vi "Write Reader.vi"(8 "error in (no error)":errorcluster, 10 "BaseReader.lvclass":refnum<class "BaseReader.lvclass">, 11 "BaseDriver in":refnum<class "BaseDriver.lvclass">) -> (0 "error out":errorcluster, 3 "BaseDriver out":refnum<class "BaseDriver.lvclass">)   [LabVIEW 2013, in "BaseDriver.lvclass"]
doc: "The Reader is the object that will perform the actual writing and reading from the remote destination. It should be a child of the BaseReader class and contains overloadded methods for writing to whatever destination it communicates with, such as a serial line or a TCP/IP connection"
uses:
  BaseDriver.lvclass
  Reader/BaseReader/BaseReader.lvclass
  BaseDriver.lvclass/BaseDriver.ctl
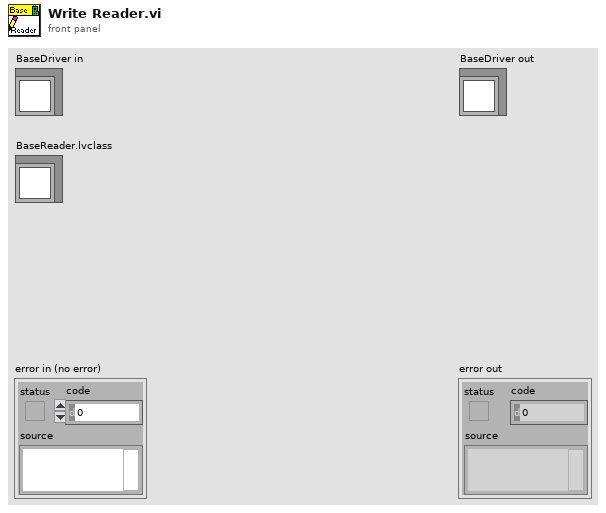
[diagram p1: front panel]
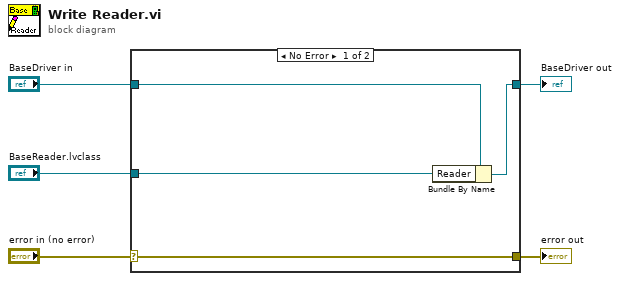
[diagram p0: block diagram]
diagram:
  n1 = case shown="No Error" "error in (no error)" {
    selector: "error in (no error)" -> [w9 w10]
    tunnel: [w9 w10] -> w4
    tunnel: [w7 w11] -> w2
    tunnel: "BaseDriver in" -> [w8 w11]
    tunnel: "BaseReader.lvclass" -> [w6 _]
    frame No Error {
      n2 = Bundle By Name(cluster=w8, "Reader"=w6) -> (w7:refnum<class "BaseDriver.lvclass">)
    }
    frame Error {
    }
  }
  "error out" <- w4
  "BaseDriver out" <- w2
